vi "GetPoint.vi"(8 "error in (no error)":errorcluster, 11 "Triangle in":refnum<class "Losange.lvclass">) -> (0 "error out":errorcluster, 2 "Point":refnum<class "Point.lvclass">, 3 "Triangle out":refnum<class "Losange.lvclass">)   [LabVIEW 2021, in "Picture2D.lvlib" / "Losange.lvclass"]
uses:
  Losange.lvclass
  Polygone/Polygone.lvclass
  Point/Point.lvclass
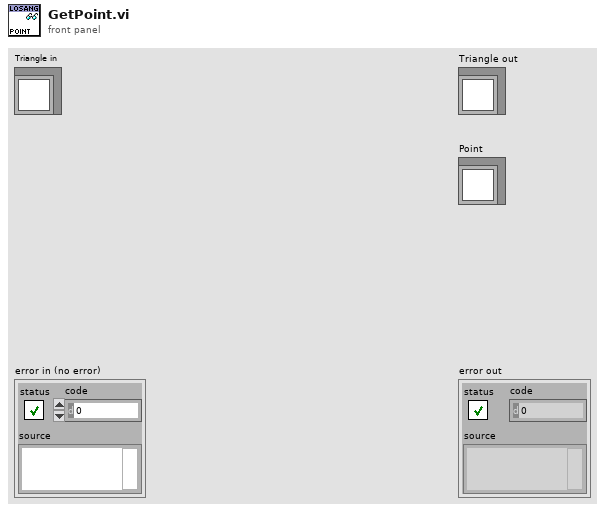
[diagram p1: front panel]
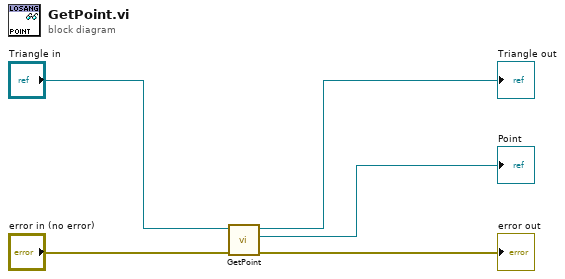
[diagram p0: block diagram]
diagram:
  n1 = call-parent "GetPoint.vi"("error in (no error)"="error in (no error)", "Picture2D in"="Triangle in") -> ("error out"=→"error out":errorcluster, "Point"=→"Point":refnum<class "Point.lvclass">, "Picture2D out"=→"Triangle out":refnum<class "Losange.lvclass">)  [unwired: 7 in]
